vi "Read Axes.vi"(0 "Arduino Resource":T1, 11 "error in (no error)":errorcluster) -> (4 "Arduino Resource":T1, 6 "X":i16, 8 "Z":i16, 10 "Y":i16, 15 "error out":errorcluster)   [LabVIEW 2012, in "Digital Compass HMC5883L.lvlib"]
uses:
  Digital Compass HMC5883L.lvlib
  <vilib>/LabVIEW Interface for Arduino/Type Defs/Arduino Resource.ctl
  <vilib>/LabVIEW Interface for Arduino/Type Defs/Board Type.ctl
  Registers.ctl
  <vilib>/LabVIEW Interface for Arduino/LabVIEW Interface for Arduino.lvlib
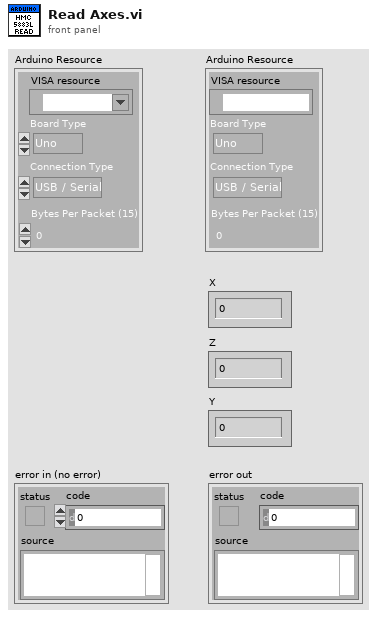
[diagram p1: front panel]
types:
  T1 = typedef "LabVIEW Interface for Arduino.lvlib/Arduino Resource.ctl" = cluster{"VISA resource":refnum<visa-resource-name>, "Board Type":T2, "Connection Type":enum8{"USB / Serial"}, "Bytes Per Packet (15)":u8}
  T2 = typedef "LabVIEW Interface for Arduino.lvlib/Board Type.ctl" = enum16{"Uno", "Dimuelanove w/Atmega 328", "Mega 2560"}
  T3 = typedef "Digital Compass HMC5883L.lvlib/Registers.ctl" = enum16{"Config A", "Config B", "Mode", "X MSB", "X LSB", "Z MSB", "Z LSB", "Y MSB", "Y LSB", "Status", "ID A", "ID B", "ID C"}
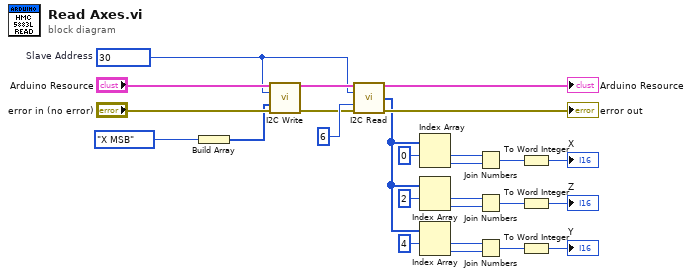
[diagram p0: block diagram]
diagram:
  w1 = u8 30  # Slave Address
  n1 = Build Array(Registers."X MSB" ("Register")) -> (w3:T3[])
  n2 = call <vilib>:"I2C Write.vi"("Arduino Resource"="Arduino Resource", "Address (0)"=w1, "I2C Data Bytes"=w3, "error in"="error in (no error)") -> ("Arduino Resource"=w5:T1, "error out"=w4:errorcluster)  [unwired: 10 in]
  n3 = call <vilib>:"I2C Read.vi"("Arduino Resource"=w5, "Address (0)"=w1, "Bytes To Read"=u8 6, "error in"=w4) -> ("Arduino Resource"=→"Arduino Resource":T1, "I2C Data"=w19:u8[], "error out"=→"error out":errorcluster)  [unwired: 9 in]
  n4 = Index Array(array=w19, index #1=0 ("index")) -> (element #1=w14:u8, element #2=w13:u8)  [unwired: 1 in]
  n5 = Index Array(array=w19, index #1=2 ("index")) -> (element #1=w15:u8, element #2=w16:u8)  [unwired: 1 in]
  n6 = Index Array(array=w19, index #1=4 ("index")) -> (element #1=w17:u8, element #2=w18:u8)  [unwired: 1 in]
  n7 = Join Numbers(hi=w14, lo=w13) -> ((hi.lo)=w22:u16)
  n8 = Join Numbers(hi=w15, lo=w16) -> ((hi.lo)=w24:u16)
  n9 = Join Numbers(hi=w17, lo=w18) -> ((hi.lo)=w26:u16)
  n10 = To Word Integer(number=w22) -> (16bit integer=→"X":i16)
  n11 = To Word Integer(number=w24) -> (16bit integer=→"Z":i16)
  n12 = To Word Integer(number=w26) -> (16bit integer=→"Y":i16)
